vi "Socket_Select.vi"(4 "error in":errorcluster, 5 "GHI":bool, 6 "DEF":bool, 7 "ABC":bool) -> (0 "error out":errorcluster, 1 "G":bool, 2 "D":bool, 3 "A":bool)   [LabVIEW 2019]
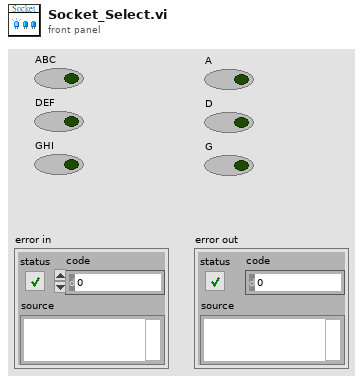
[diagram p1: front panel]
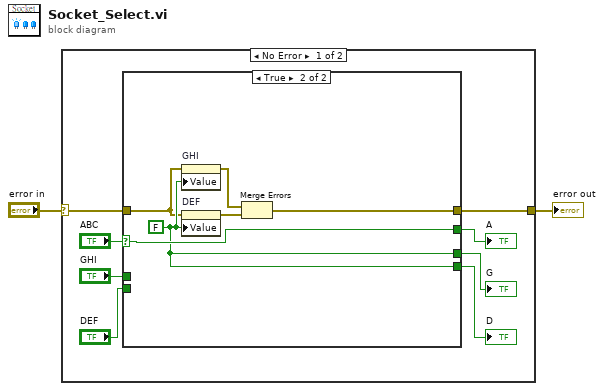
[diagram p0: block diagram]
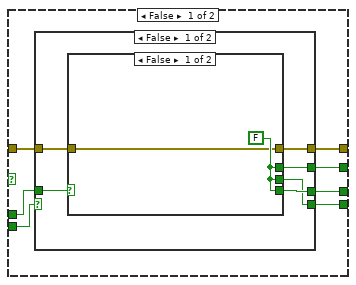
[diagram p2: hidden frame]
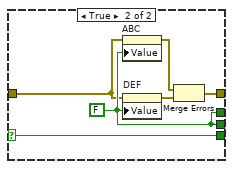
[diagram p3: hidden frame]
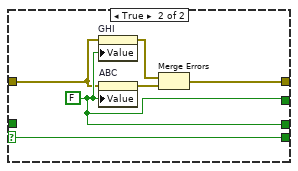
[diagram p4: hidden frame]
diagram:
  n1 = case shown="No Error" "error in" {
    selector: "error in" -> [w4 w44]
    tunnel: [w3 w44] -> w1
    frame No Error {
      n2 = case shown="True" "ABC" {
        selector: "ABC" -> [_ w43]
        tunnel: [w15 w43] -> w6
        tunnel: [w16 w42] -> w7
        tunnel: [w14 w42] -> w8
        tunnel: "DEF" -> [w17 _]
        tunnel: "GHI" -> [w13 _]
        tunnel: w4 -> [w12 w41]
        tunnel: [w11 w38] -> w3
        frame False {
          n3 = case shown="False" w17 {
            selector: w17 -> [_ w37]
            tunnel: [w20 w37] -> w16
            tunnel: [w21 w36] -> w15
            tunnel: [w22 w36] -> w14
            tunnel: w13 -> [w23 _]
            tunnel: w12 -> [w19 w35]
            tunnel: [w18 w32] -> w11
            frame False {
              n4 = case shown="False" w23 {
                selector: w23 -> [_ w31]
                tunnel: [w25 w31] -> w22
                tunnel: [w25 w30] -> w21
                tunnel: [w25 w30] -> w20
                tunnel: w19 -> [w24 w27]
                tunnel: [w24 w28] -> w18
                frame False {
                  w25 = FALSE
                }
                frame True {
                  w30 = FALSE
                  n5 = property on="ABC" class="Bool (strict)"(error in=w27, "Value"=w30) -> (error out=w29:errorcluster)  [unwired: 1 in, 1 out]
                  n6 = property on="DEF" class="Bool (strict)"(error in=w27, "Value"=w30) -> (error out=w26:errorcluster)  [unwired: 1 in, 1 out]
                  n7 = Merge Errors(w29, w26) -> (w28:errorcluster)
                }
              }
            }
            frame True {
              w36 = FALSE
              n8 = property on="GHI" class="Bool (strict)"(error in=w35, "Value"=w36) -> (error out=w34:errorcluster)  [unwired: 1 in, 1 out]
              n9 = property on="ABC" class="Bool (strict)"(error in=w35, "Value"=w36) -> (error out=w33:errorcluster)  [unwired: 1 in, 1 out]
              n10 = Merge Errors(w34, w33) -> (w32:errorcluster)
            }
          }
        }
        frame True {
          w42 = FALSE
          n11 = property on="GHI" class="Bool (strict)"(error in=w41, "Value"=w42) -> (error out=w40:errorcluster)  [unwired: 1 in, 1 out]
          n12 = property on="DEF" class="Bool (strict)"(error in=w41, "Value"=w42) -> (error out=w39:errorcluster)  [unwired: 1 in, 1 out]
          n13 = Merge Errors(w40, w39) -> (w38:errorcluster)
        }
      }
      "G" <- w8
      "D" <- w7
      "A" <- w6
    }
    frame Error {
    }
  }
  "error out" <- w1
